vi "CloseDevice.vi"(8 "error in (no error)":errorcluster, 11 "id":u16) -> (0 "错误输出":errorcluster)   [LabVIEW 2011]
panel:
  out "返回类型":i32
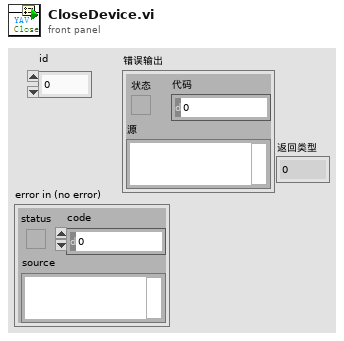
[diagram p1: front panel]
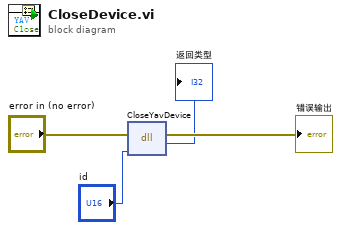
[diagram p0: block diagram]
diagram:
  n1 = dll-call lib="PTH1abs Eäº§åç å åªé³-Labviewï¼è¯ç­æµè¯ï¼,åªé³labviewï¼è¯ç­æµè¯ï¼ YAVééå¡UMS å¼æºä¾ç¨LabVIEW 2017data\nADIO86.dll" fn="CloseYavDevice"(error in="error in (no error)", "ID"="id") -> (error out=→"错误输出":errorcluster, "返回类型"=→"返回类型":i32)  [unwired: 3 in, 1 out]
